vi "value to ring (StartMode).vi"(11 "value":string) -> (3 "StartMode":i32)   [LabVIEW 2020, in "AIM ARINC 664 Import.lvlib"]
uses:
  AIM ARINC 664 Import.lvlib
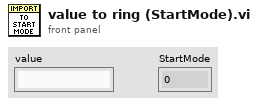
[diagram p1: front panel]
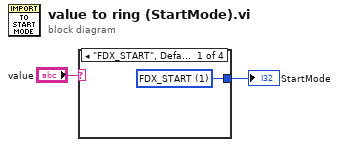
[diagram p0: block diagram]
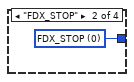
[diagram p2: hidden frame]
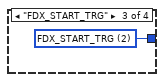
[diagram p3: hidden frame]
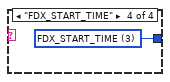
[diagram p4: hidden frame]
diagram:
  n1 = case shown="\"FDX_START\", Default" "value" {
    tunnel: [w3 w4 w5 w6] -> w1
    frame "FDX_START", Default {
      w3 = 1 items=["FDX_STOP", "FDX_START", "FDX_START_TRG", "FDX_START_TIME"] ("StartMode")
    }
    frame "FDX_STOP" {
      w4 = 0 items=["FDX_STOP", "FDX_START", "FDX_START_TRG", "FDX_START_TIME"] ("StartMode")
    }
    frame "FDX_START_TRG" {
      w5 = 2 items=["FDX_STOP", "FDX_START", "FDX_START_TRG", "FDX_START_TIME"] ("StartMode")
    }
    frame "FDX_START_TIME" {
      w6 = 3 items=["FDX_STOP", "FDX_START", "FDX_START_TRG", "FDX_START_TIME"] ("StartMode")
    }
  }
  "StartMode" <- w1
